vi "keeperTarget.vi"(11 "Game in":refnum<class "Game.lvclass">) -> (2 "pass":bool=TRUE, 3 "target":dbl[](array[numeric]))   [LabVIEW 2024, in "DefendGoalTactic.lvclass"]
uses:
  DefendGoalTactic.lvclass
  Game_class/Game.lvclass
  Robot_class/roles.ctl
  Game_class/Game.lvclass/Game.ctl
  Team_class/Team.lvclass/Team.ctl
  Object_class/Object.lvclass/Object.ctl
  Parameters_class/Parameters.lvclass/Parameters.ctl
  Game_class/Read FieldRef.vi
  Game_class/Read Utilities.lvclass.vi
  Game_class/Read Parameters.lvclass.vi
  Parameters_class/Read AttakingOurselves.vi
  Object_class/Read x.vi
  Object_class/Read y.vi
  Game_class/Read OffensiveTeam.vi
  Team_class/Read RobotRef.vi
  Ally_class/Ally.lvclass
  C:/Users/ROBOIME2/Documents/SSL ROBOIME/SSL_AI/Team_class/Team.lvclass
  Robot_class/Robot.lvclass
  C:/Users/ROBOIME2/Documents/SSL ROBOIME/SSL_AI/Object_class/Object.lvclass
  Field_class/Field.lvclass
  Utilities_class/Utilities.lvclass
  Parameters_class/Parameters.lvclass
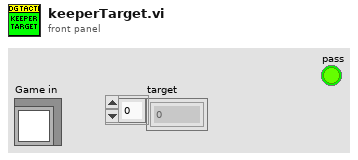
[diagram p1: front panel]
types:
  T1 = typedef "roles.ctl" = enum16{"SimpleBallPlacement", "BallPlacementAllyPasser", "BallPlacementAllyReceiver", "BallPlacementEnemy", "5Robots5th", "PassBestReceiver", "5Robots4th", "5Robots3rd", "5Robots2nd", "5Robots1st", "PassBestRobot", "WaitPass", "ABCThirdKicker", "ABCFirstKicker", "ABCSecondKicker", "Tabler", "TableFinalizer", "PrepareRollToPassRoller", "PrepareRollToPassReceiver", "SimplePassRoll", "SimplePassRollReceiver", "PenaltyDefense", "PreparePassReceiver 2", "PreparePassReceiver 1", "PassObserver", "Timeout", "Goto", "ZigZag", "None", "BallOutOfField", "DefenderArea", "Duelist", "AttackerStop", "FollowAttacker", "KeeperRole", "KickPenalty", "AttackerAimGoal", "AttackerBlock", "Marker", "Halt", "Shoot", "PassKicker", "PassReceiver", "TestRole", "PenaltyAttacker"}
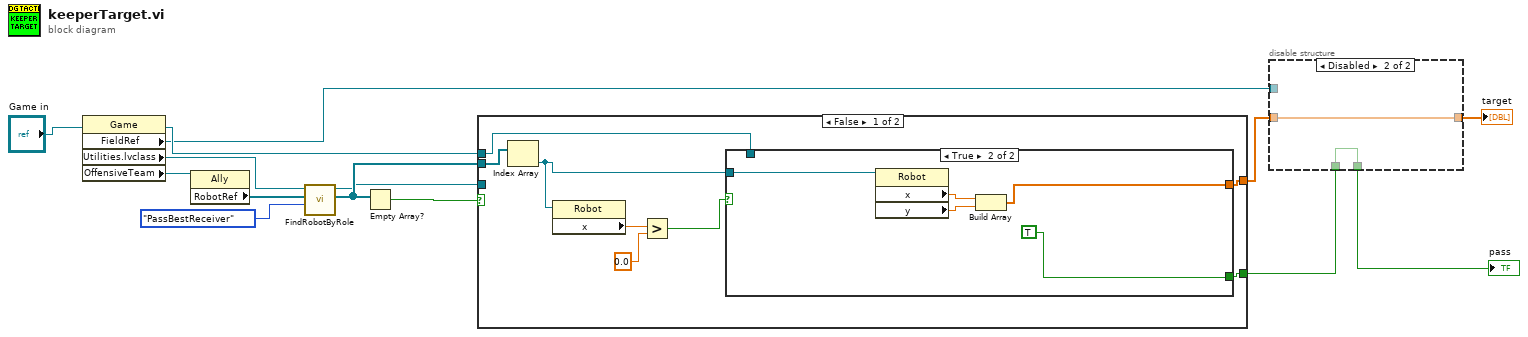
[diagram p0: block diagram]
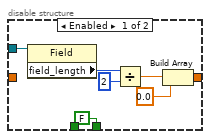
[diagram p2: hidden frame]
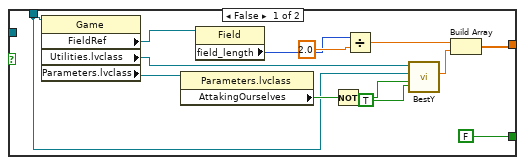
[diagram p3: hidden frame]
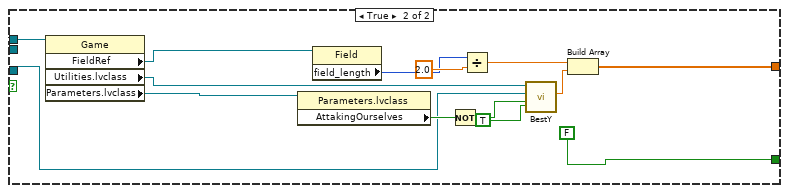
[diagram p4: hidden frame]
diagram:
  n1 = property class="Game"(reference="Game in") -> ("FieldRef"=w5:refnum<class "Field.lvclass">, "Utilities.lvclass"=w10:refnum<class "Utilities.lvclass">, "OffensiveTeam"=w12:refnum<class "Ally.lvclass">)  [unwired: 1 in, 2 out]
  n2 = property class="Ally"(reference=w12) -> ("RobotRef"=w11:refnum<class "Robot.lvclass">[])  [unwired: 1 in, 2 out]
  n3 = call "FindRobotByRole.vi"("role"=roles."PassBestReceiver", "RobotRef"=w11, "Utilities in"=w10) -> ("Robots"=w7:refnum<class "Robot.lvclass">[], "Utilities out"=w6:refnum<class "Utilities.lvclass">)  [unwired: 5 in, 2 out]
  n4 = Empty Array?(array=w7) -> (empty?=w8:bool)
  n5 = case shown="False" w8 {
    tunnel: [w20 w47] -> w2
    tunnel: "Game in" -> [w18 w42]
    tunnel: w7 -> [w21 _]
    tunnel: [w19 FALSE] -> w1
    tunnel: w6 -> [_ _]
    frame False {
      n6 = Index Array(array=w21) -> (element=w17:refnum<class "Robot.lvclass">)  [unwired: 1 in]
      n7 = property class="Robot"(reference=w17) -> ("x"=w16:dbl)  [unwired: 1 in, 2 out]
      n8 = Greater?(x=w16, y=0.0) -> (0:w15:bool)
      n9 = case shown="True" w15 {
        tunnel: [w22 w37] -> w20
        tunnel: w17 -> [_ w36]
        tunnel: [FALSE TRUE] -> w19
        tunnel: w18 -> [w24 _]
        frame False {
          n10 = property class="Game"(reference=w24) -> ("FieldRef"=w30:refnum<class "Field.lvclass">, "Utilities.lvclass"=w25:refnum<class "Utilities.lvclass">, "Parameters.lvclass"=w26:refnum<class "Parameters.lvclass">)  [unwired: 1 in, 2 out]
          n11 = property class="Parameters.lvclass"(reference=w26) -> ("AttakingOurselves"=w28:bool)  [unwired: 1 in, 2 out]
          n12 = property class="Field"(reference=w30) -> ("field_length"=w31:i32)  [unwired: 1 in, 2 out]
          n13 = Not(x=w28) -> (.not. x?=w27:bool)
          n14 = Divide(x=w31, y=2.0) -> (x/y=w33:dbl)
          n15 = call "BestY.vi"("Utilities in"=w25, "Game"=w24, "inimigos"=w27, "Goalie?"=TRUE) -> ("Best y"=w29:dbl)  [unwired: 1 in, 4 out]
          n16 = Build Array(w33, w29) -> (w22:dbl[])
        }
        frame True {
          n17 = property class="Robot"(reference=w36) -> ("x"=w39:dbl, "y"=w38:dbl)  [unwired: 1 in, 2 out]
          n18 = Build Array(w39, w38) -> (w37:dbl[])
        }
      }
    }
    frame True {
      n19 = property class="Game"(reference=w42) -> ("FieldRef"=w48:refnum<class "Field.lvclass">, "Utilities.lvclass"=w41:refnum<class "Utilities.lvclass">, "Parameters.lvclass"=w43:refnum<class "Parameters.lvclass">)  [unwired: 1 in, 2 out]
      n20 = property class="Parameters.lvclass"(reference=w43) -> ("AttakingOurselves"=w45:bool)  [unwired: 1 in, 2 out]
      n21 = property class="Field"(reference=w48) -> ("field_length"=w49:i32)  [unwired: 1 in, 2 out]
      n22 = Not(x=w45) -> (.not. x?=w44:bool)
      n23 = Divide(x=w49, y=2.0) -> (x/y=w51:dbl)
      n24 = call "BestY.vi"("Utilities in"=w41, "Game"=w42, "inimigos"=w44, "Goalie?"=TRUE) -> ("Best y"=w46:dbl)  [unwired: 1 in, 4 out]
      n25 = Build Array(w51, w46) -> (w47:dbl[])
    }
  }
  n26 = disable-structure shown="Disabled" {
    disable-tunnel: w5 -> [w59 _]
    disable-tunnel: [w54 w61] -> w4
    disable-tunnel: [FALSE ("pass") w60] -> w3
    disable-tunnel: w2 -> [_ w61]
    disable-tunnel: w1 -> [_ w60]
    frame Enabled {
      n27 = property class="Field"(reference=w59) -> ("field_length"=w58:i32)  [unwired: 1 in, 2 out]
      n28 = Divide(x=w58, y=2) -> (x/y=w56:dbl)
      n29 = Build Array(w56, 0.0 ("element")) -> (w54:dbl[])
    }
    frame Disabled {
    }
  }
  "target" <- w4
  "pass" <- w3
